vi "Unknown MSG Received from Host--error.vi"(10 "Data":string, 11 "Command":string) -> (0 "error out":errorcluster)   [LabVIEW 2021, in "RT Interpreter Manager.lvlib"]
uses:
  RT Interpreter Manager.lvlib
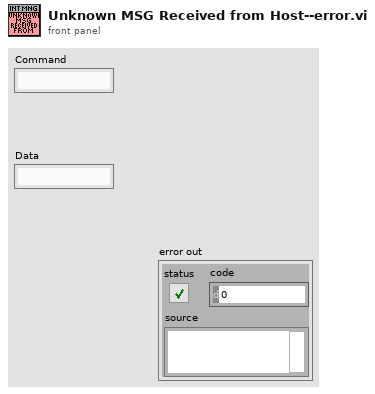
[diagram p1: front panel]
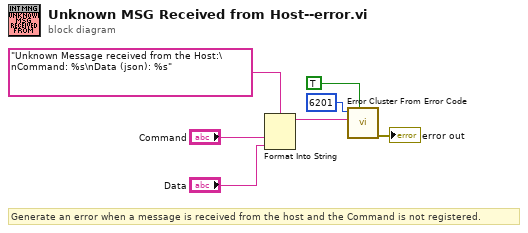
[diagram p0: block diagram]
diagram:
  # "Generate an error when a message is received from the host and the Command is not registered."
  n1 = Format Into String(format string="Unknown Message received from the Host:\nCommand: %s\nData (json): %s", "Command", "Data") -> (resulting string=w1:string)  [unwired: 2 in, 1 out]
  n2 = call <vilib>:"Error Cluster From Error Code.vi"("show call chain? (False)"=TRUE, "error message (\"\")"=w1, "error code (0)"=6201) -> ("error out"=→"error out":errorcluster)  [unwired: 6 in]
